vi "Write Channels.vi"(8 "error in (no error)":errorcluster, 10 "Channels":T1[](array[typedef]), 11 "DCM-DSI-HW in":refnum<class "DCM-DSI.lvclass">) -> (0 "error out":errorcluster, 3 "DCM-DSI-HW out":refnum<class "DCM-DSI.lvclass">)   [LabVIEW 2016, in "DCM-DSI.lvclass"]
uses:
  DCM-DSI.lvclass
  Shared/Typedefs/Engine-Channel.ctl
  DCM-DSI.lvclass/DCM-DSI.ctl
  Shared/DSI-Shared.lvlib
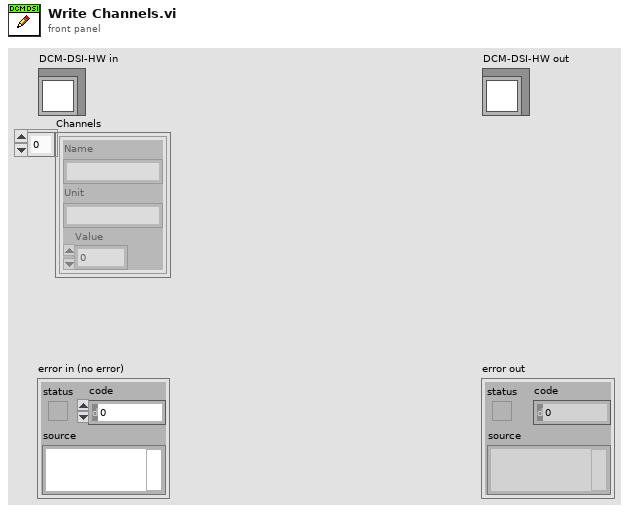
[diagram p1: front panel]
types:
  T1 = typedef "DSI-Shared.lvlib/Engine-Channel.ctl" = cluster{"Name":string, "Unit":string, "Value":sgl}
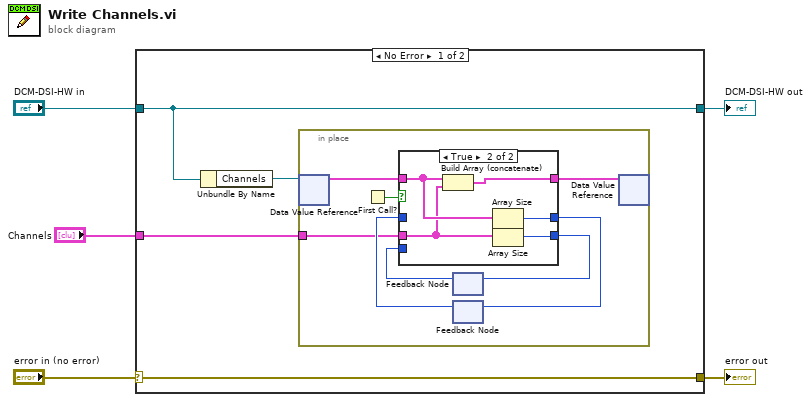
[diagram p0: block diagram]
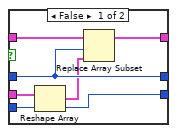
[diagram p2: hidden frame]
diagram:
  n1 = case shown="No Error" "error in (no error)" {
    selector: "error in (no error)" -> [w9 w30]
    tunnel: [w9 w30] -> w4
    tunnel: [w7 w29] -> w2
    tunnel: "DCM-DSI-HW in" -> [w7 w29]
    tunnel: "Channels" -> [w6 _]
    frame No Error {
      n2 = Unbundle By Name(w7) -> ("Channels"=w8:refnum<data-value>)
      n3 = in-place {
        in-place-border: w6 -> [w11]
        n4 = in-place-dvr #1(w8) -> (w13:T1[])  [unwired: 1 out]
        n5 = First Call?() -> (First Call?: T/F=w10:bool)
        n6 = feedback #2() -> (w16:i32)  [unwired: 1 in]
        n7 = feedback #3() -> (w17:i32)  [unwired: 1 in]
        n8 = case shown="True" w10 {
          tunnel: w13 -> [w23 w26]
          tunnel: w11 -> [w20 w25]
          tunnel: [w22 w28] -> w12
          tunnel: [w21 w27] -> w14
          tunnel: w17 -> [w21 _]
          tunnel: [w18 w24] -> w15
          tunnel: w16 -> [w18 _]
          frame False {
            n9 = Reshape Array(w20, w18) -> (w19:T1[])
            n10 = Replace Array Subset(array=w23, new element=w19, index=w21) -> (w22:T1[])
          }
          frame True {
            n11 = Build Array (concatenate)(w26, w25) -> (w28:T1[])
            n12 = Array Size(array=w26) -> (size(s)=w27:i32)
            n13 = Array Size(array=w25) -> (size(s)=w24:i32)
          }
        }
        n14 = feedback-in #2(w15) -> ()
        n15 = feedback-in #3(w14) -> ()
        n16 = in-place-dvr #1(w12) -> ()  [unwired: 2 out]
      }
    }
    frame Error {
    }
  }
  "error out" <- w4
  "DCM-DSI-HW out" <- w2
